vi "New Step at End.vi"(8 "error in (no error)":errorcluster, 9 "PanelArray":refnum<class "PanelArray.lvclass">, 10 "Step Type":T1, 11 "Recipe Editor in":refnum<class "Recipe Editor.lvclass">) -> (0 "error out":errorcluster, 3 "Recipe Editor out":refnum<class "Recipe Editor.lvclass">)   [LabVIEW 2018, in "Temp Recipe.lvlib" / "Recipe Editor.lvclass"]
uses:
  Recipe Editor.lvclass
  Step Type.ctl
  Libraries/OOPanel/OOPanel/PanelArray/PanelArray.lvclass
  Recipe Editor.lvclass/Recipe Editor.ctl
  Recipe Step/Recipe Step.lvclass
  C:/dev/source/Libraries/OOPanel/OOPanel/Panel/Panel.lvclass
  Libraries/OOPanel/OOPanel/Panel/Panel.lvclass
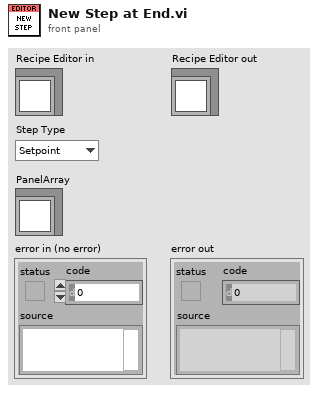
[diagram p1: front panel]
types:
  T1 = typedef "Temp Recipe.lvlib/Recipe Editor.lvclass/Step Type.ctl" = enum16{"Setpoint", "Step Rate", "Rate Duration", "Delay"}
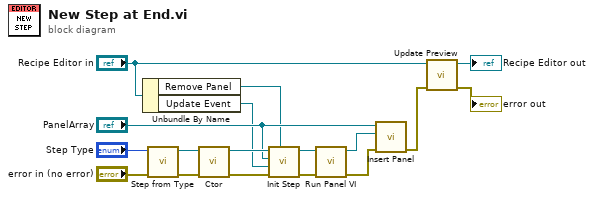
[diagram p0: block diagram]
diagram:
  n1 = Unbundle By Name("Recipe Editor in") -> ("Remove Panel"=w1:refnum<user-event>, "Update Event"=w6:refnum<user-event>)
  n2 = call "Step from Type.vi"("Step Type"="Step Type") -> ("Step"=w15:refnum<class "Recipe Step.lvclass">)  [unwired: 10 in]
  n3 = call-dynamic "Ctor.vi"("error in (no error)"="error in (no error)", "Panel in"=w15) -> ("error out"=w9:errorcluster, "Panel out"=w10:refnum<class "Recipe Step.lvclass">)  [unwired: 8 in]
  n4 = call "Init Step.vi"("Remove Panel"=w1, "error in (no error)"=w9, "Update Event"=w6, "PanelArray"="PanelArray", "Recipe Step in"=w10) -> ("error out"=w4:errorcluster, "Recipe Step out"=w5:refnum<class "Recipe Step.lvclass">)  [unwired: 5 in]
  n5 = call "Run Panel VI.vi"("error in (no error)"=w4, "Panel in"=w5) -> ("error out"=w2:errorcluster, "Panel out"=w3:refnum<class "Recipe Step.lvclass">)  [unwired: 8 in]
  n6 = call "Insert Panel.vi"("error in (no error)"=w2, "Panel In"=w3, "PanelArray in"="PanelArray") -> ("error out"=w12:errorcluster)  [unwired: 7 in, 1 out]
  n7 = call "Update Preview.vi"("error in (no error)"=w12, "Recipe Editor in"="Recipe Editor in") -> ("error out"=→"error out":errorcluster, "Recipe Editor out"=→"Recipe Editor out":refnum<class "Recipe Editor.lvclass">)  [unwired: 8 in]
